vi "Inst.FP.ParseGHSmode.vi"(3 "GHS.Mode":u16) -> (0 "mode string":string, 1 "mode enum":T1)   [LabVIEW 2019, in "Inst.FP.lvclass"]
uses:
  Inst.FP.lvclass
  Typedefs/Inst.FP.Modes--Enum.ctl
  <userlib>/LevyLab/Instrument Framework/SMOs/Instrument/Instrument.lvclass
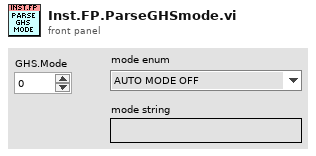
[diagram p1: front panel]
types:
  T1 = typedef "Inst.FP.lvclass/Inst.FP.Modes--Enum.ctl" = enum16{"AUTO MODE OFF", "START", "CONDENSING 3He", "CONDENSING 4He", "NORMAL CIRCULATION", "RECOVERY OF THE MIXTURE", "RECOVERY: BLOCKAGE or OVERPRESSURE"}
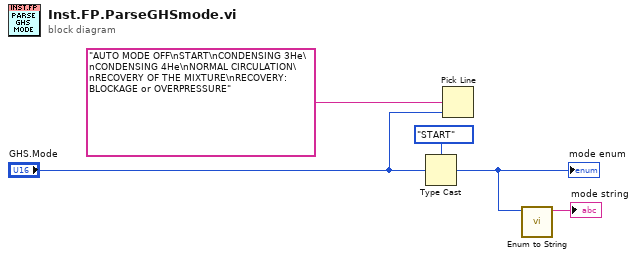
[diagram p0: block diagram]
diagram:
  n1 = Type Cast(type=Inst.FP.Modes--Enum."START" ("Mode"), x="GHS.Mode") -> (*(type *) &x=w1:T1)
  "mode enum" <- w1
  n2 = Pick Line(multi-line string="AUTO MODE OFF\nSTART\nCONDENSING 3He\nCONDENSING 4He\nNORMAL CIRCULATION\nRECOVERY OF THE MIXTURE\nRECOVERY: BLOCKAGE or OVERPRESSURE", line index="GHS.Mode") -> ()  [unwired: 1 in, 1 out]
  n3 = call <userlib>:"Enum to String.vi"("Command"=w1) -> ("Command"=→"mode string":string)  [unwired: 9 in, 1 out]
